vi "get_next.vi"(8 "error in (no error)":errorcluster, 11 "DoublyNodeRef in":refnum<class "Iterator.lvclass">) -> (0 "error out":errorcluster, 1 "found?":bool, 2 "next":refnum<class "Iterator.lvclass">, 3 "DoublyNodeRef out":refnum<class "Iterator.lvclass">)   [LabVIEW 2021, in "Iterator.lvclass"]
uses:
  Iterator.lvclass
  Iterator.lvclass/Iterator.ctl
  IDoublyNode/IDoublyNode.lvclass
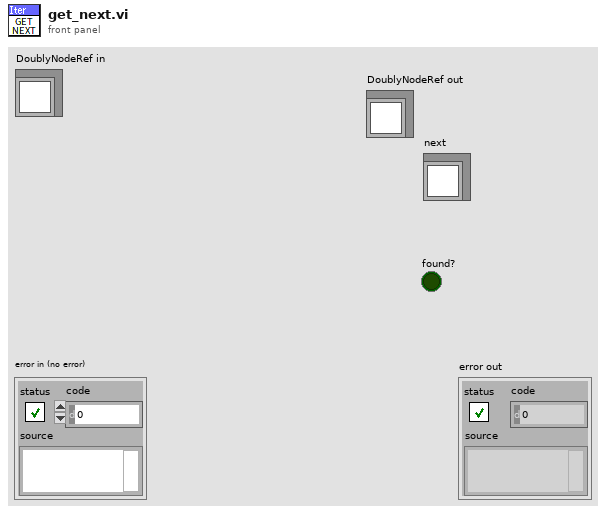
[diagram p1: front panel]
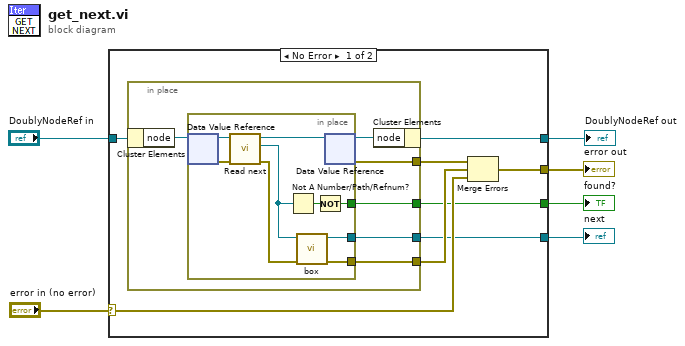
[diagram p0: block diagram]
diagram:
  n1 = case shown="No Error" "error in (no error)" {
    selector: "error in (no error)" -> [w13 w31]
    tunnel: [w12 w31] -> w5
    tunnel: "DoublyNodeRef in" -> [w14 w30]
    tunnel: [w9 _] -> w2
    tunnel: [w8 _] -> w3
    tunnel: [w7 w30] -> w1
    frame No Error {
      n2 = in-place {
        in-place-border: [w18] -> w8
        in-place-border: [w17] -> w10
        in-place-border: [w16] -> w11
        in-place-border: [w15] -> w9
        n3 = in-place-cluster #1(w14) -> ("node"=w20:refnum<data-value>)
        n4 = in-place {
          in-place-border: [w25] -> w18
          in-place-border: [w24] -> w17
          in-place-border: [w21] -> w15
          n5 = in-place-dvr #2(w20) -> (w29:refnum<class "IDoublyNode.lvclass">, w27:errorcluster)
          n6 = call-dynamic "Read next.vi"("error in (no error)"=w27, "NodeType in"=w29) -> ("error out"=w26:errorcluster, "next"=w23:refnum<data-value>, "NodeType out"=w28:refnum<class "IDoublyNode.lvclass">)  [unwired: 7 in]
          n7 = Not A Number/Path/Refnum?(number/path/refnum=w23) -> (NaN/Path/Refnum?=w22:bool)
          n8 = call "box.vi"("error in (no error)"=w26, "node"=w23) -> ("error out"=w24:errorcluster, "DoublyNodeRef out"=w25:refnum<class "Iterator.lvclass">)  [unwired: 8 in]
          n9 = Not(x=w22) -> (.not. x?=w21:bool)
          n10 = in-place-dvr #2(w28) -> (w19:refnum<data-value>, w16:errorcluster)
        }
        n11 = in-place-cluster #1("node"=w19) -> (w7:refnum<class "Iterator.lvclass">)
      }
      n12 = Merge Errors(w11, w10, w13) -> (w12:errorcluster)
    }
    frame Error {
    }
  }
  "error out" <- w5
  "next" <- w3
  "found?" <- w2
  "DoublyNodeRef out" <- w1
